vi "niFPGA Handshake Pipe Stage Logic.vi"(9 "last output valid":bool, 11 "ready for output":bool) -> (3 "ready For input":bool)   [LabVIEW 2017]
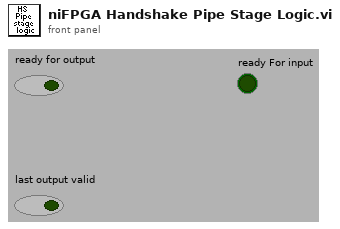
[diagram p1: front panel]
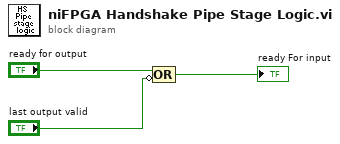
[diagram p0: block diagram]
diagram:
  n1 = Compound Arithmetic op=OR("ready for output", invert "last output valid") -> (→"ready For input":bool)
